vi "ListVILibraryCalls.vi"(8 "error in (no error)":errorcluster, 11 "VI Refnum":refnum<vi>) -> (0 "error out":errorcluster, 2 "VI Call Library Nodes":refnum<vi>[](array[refnum]))   [LabVIEW 2024, in "Scripts.lvlib"]
uses:
  Scripts.lvlib
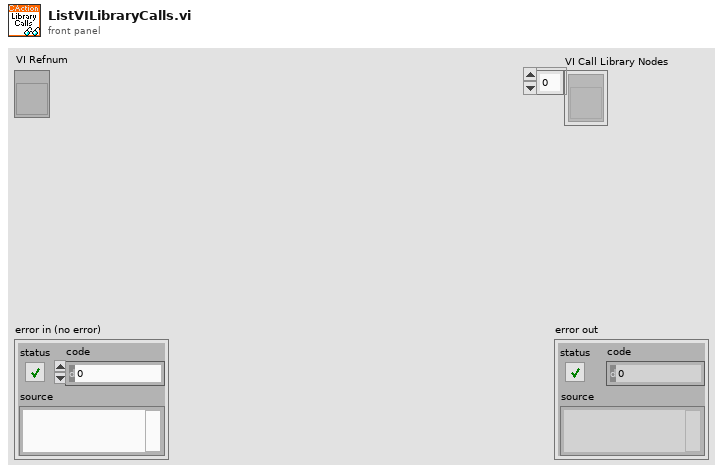
[diagram p1: front panel]
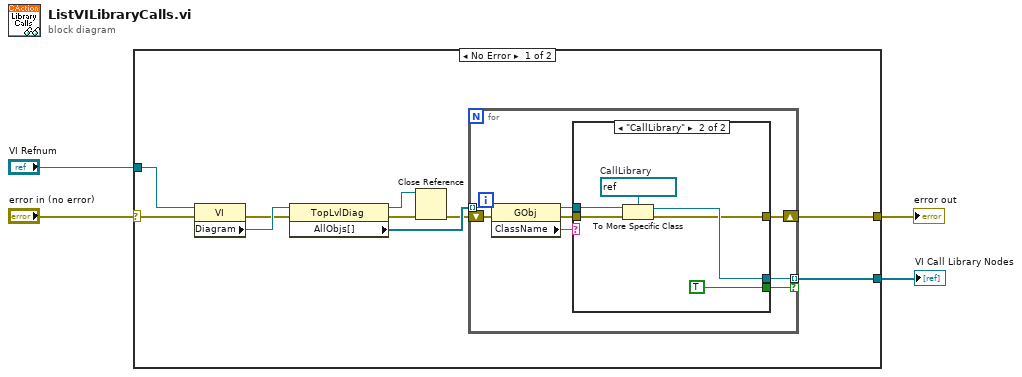
[diagram p0: block diagram]
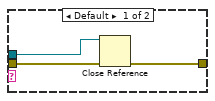
[diagram p2: hidden frame]
diagram:
  n1 = case shown="No Error" "error in (no error)" {
    selector: "error in (no error)" -> [w9 w32]
    tunnel: "VI Refnum" -> [w14 _]
    tunnel: [w5 w32] -> w2
    tunnel: [w8 _] -> w1
    frame No Error {
      n2 = property class="VI"(reference=w14, error in=w9) -> (error out=w12:errorcluster, "Diagram"=w13:refnum<vi>)  [unwired: 1 out]
      n3 = property class="TopLvlDiag"(reference=w13, error in=w12) -> (reference out=w6:refnum<vi>, error out=w11:errorcluster, "AllObjs[]"=w10:refnum<vi>[])
      n4 = Close Reference(reference=w6, error in (no error)=w11) -> (error out=w7:errorcluster)
      n5 = for {
        tunnel: w10 -> [w21] mode=indexing
        shift-right: [w19] -> w5
        shift-left: w7 -> [w22]
        tunnel: [w16] -> w8 mode=indexing if=w15
        n6 = property class="GObj"(reference=w21, error in=w22) -> (reference out=w18:refnum<vi>, error out=w20:errorcluster, "ClassName"=w17:string)
        n7 = case shown="\"CallLibrary\"" w17 {
          tunnel: w20 -> [w25 w31]
          tunnel: [w24 w27] -> w19
          tunnel: w18 -> [w23 w30]
          tunnel: [_ w28] -> w16
          tunnel: [_ TRUE] -> w15
          frame Default {
            n8 = Close Reference(reference=w23, error in (no error)=w25) -> (error out=w24:errorcluster)
          }
          frame "CallLibrary" {
            w29 = refnum<vi> refnum  # CallLibrary
            n9 = To More Specific Class(target class=w29, reference=w30, error in=w31) -> (specific class reference=w28:refnum<vi>, error out=w27:errorcluster)
          }
        }
      }
    }
    frame Error {
    }
  }
  "error out" <- w2
  "VI Call Library Nodes" <- w1
